vi "Status Reg B.vi"(1 "Status:Register:B":i16) -> (0 "Reg B":i16[](array[numeric]))   [LabVIEW 2019, in "DeltaPSControl Engine.lvlib"]
uses:
  DeltaPSControl Engine.lvlib
panel:
  out "Wait Trig":bool
  out "Prog. RUN":bool
  out "Rem CV":bool
  out "Rem CC":bool
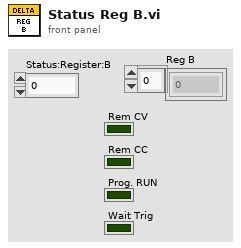
[diagram p1: front panel]
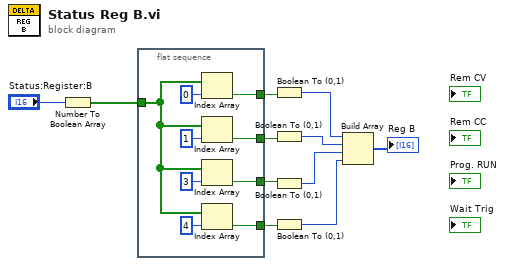
[diagram p0: block diagram]
diagram:
  n1 = Number To Boolean Array(number="Status:Register:B") -> (Boolean array=w11:bool[])
  n2 = flat-sequence {
    tunnel: w11 -> [w14]
    tunnel: [w18] -> w6
    tunnel: [w17] -> w9
    tunnel: [w13] -> w8
    tunnel: [w12] -> w7
    frame #0 {
      n3 = Index Array(array=w14, index=0) -> (element=w18:bool)
      n4 = Index Array(array=w14, index=1) -> (element=w17:bool)
      n5 = Index Array(array=w14, index=3) -> (element=w13:bool)
      n6 = Index Array(array=w14, index=4) -> (element=w12:bool)
    }
  }
  n7 = Boolean To (0,1)(Boolean=w6) -> (0, 1=w5:i16)
  n8 = Boolean To (0,1)(Boolean=w9) -> (0, 1=w4:i16)
  n9 = Boolean To (0,1)(Boolean=w8) -> (0, 1=w3:i16)
  n10 = Boolean To (0,1)(Boolean=w7) -> (0, 1=w2:i16)
  n11 = Build Array(w5, w4, w3, w2) -> (→"Reg B":i16[])
